vi "Difference Quotient (multiple).vi"(6 "Interval Units (points)":enum16{"Points", "Data"}(ring), 8 "error in (no error)":errorcluster, 9 "Type":enum16{"y/x vs x", "x/y vs y"}(ring), 10 "Window [h] (2)":dbl=2.0 min=2.0, 11 "XY-data":cluster{"X-array":dbl[], "Y-array":dbl[]}[](array[cluster]) {"Y-array" format="%.2p"; "X-array" format="%.2p"}) -> (0 "error out":errorcluster, 2 "Difference Quotient":cluster{"X-array":dbl[], "Y-array":dbl[]}[](array[cluster]), 3 "XY-data out":cluster{"X-array":dbl[], "Y-array":dbl[]}[](array[cluster]) {"Y-array" format="%.2p"; "X-array" format="%.2p"})   [LabVIEW 2016, in "xy_utilities.lvlib"]
doc: "Calculate the difference quotient (y[i-h/2]-y[i+h/s])/(x[i-h/2]-x[i+h/2]).\n\nWire data to the data input to determine the polymorphic instance to use or manually select the instance."
uses:
  xy_utilities.lvlib
  Swap X and Y.vi
  Swap X and Y (single).vi
  Private/DQ subVI.vi
  Reverse.vi
  Reverse (single).vi
  Divide.vi
  Divide float (single).vi
  Add.vi
  Add XY (single).vi
  Private/h.vi
  Private/X Array Range to Index.vi
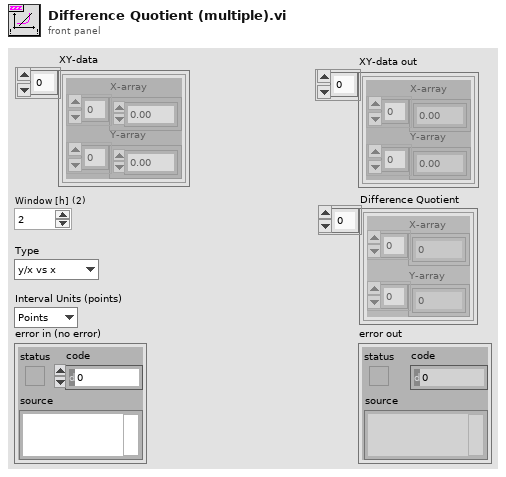
[diagram p1: front panel]
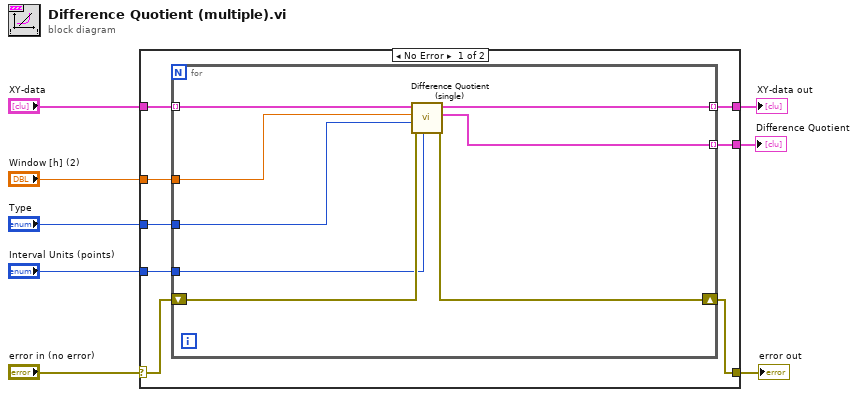
[diagram p0: block diagram]
diagram:
  n1 = case shown="No Error" "error in (no error)" {
    selector: "error in (no error)" -> [w14 w26]
    tunnel: [w13 w26] -> w7
    tunnel: "XY-data" -> [w16 w25]
    tunnel: [w15 w25] -> w5
    tunnel: "Type" -> [w12 _]
    tunnel: "Window [h] (2)" -> [w11 _]
    tunnel: [w10 _] -> w2
    tunnel: "Interval Units (points)" -> [w9 _]
    frame No Error {
      n2 = for {
        tunnel: w16 -> [w24] mode=indexing
        tunnel: [w23] -> w15 mode=indexing
        shift-right: [w20] -> w13
        shift-left: w14 -> [w21]
        tunnel: w12 -> [w17]
        tunnel: w11 -> [w19]
        tunnel: [w22] -> w10 mode=indexing
        tunnel: w9 -> [w18]
        n3 = call "Difference Quotient (single).vi"("Interval Units (points)"=w18, "error in (no error)"=w21, "Type"=w17, "Window [h] (2)"=w19, "XY-data"=w24) -> ("error out"=w20:errorcluster, "Difference Quotient"=w22:cluster{"X-array":dbl[], "Y-array":dbl[]}, "XY-data out"=w23:cluster{"X-array":dbl[], "Y-array":dbl[]})  [unwired: 4 in]
      }
    }
    frame Error {
    }
  }
  "error out" <- w7
  "XY-data out" <- w5
  "Difference Quotient" <- w2
